vi "Main.vi"() -> ()   [LabVIEW 2015]
doc: "This template is for the Queued Message Handler design pattern.\n\nThe Event Handling Loop generates messages based on user interface actions.\n\nThe Message Handling Loop processes messages generated by the Event Handling Loop, or by other messages. The messages are string values, so new messages can be added easily to the Message Cases case structure in the Message Handling Loop. Each message cluster can also provide an optional value for Message Data, which is a variant that can be converted to whatever message-specific data is required."
uses:
  support/Type Definitions/UI Data.ctl
  support/Status Logger/Status Log.ctl
  TCP/TypeDefs/TCP Data.ctl
  <vilib>/Utility/error.llb/DialogType.ctl
  DAQ/TypeDefs/DAQ data.ctl
  support/Message Queue/Enqueue Message (Single).vi
  support/Global names.vi
  <vilib>/Utility/error.llb/Error Cluster From Error Code.vi
  <vilib>/ErrorRing/Error Ring.xnode
  support/Message Queue/Message Queue.lvlib
  Support/User Event - EHL Stop/User Event - EHL Stop.lvlib
  Model/Model.lvlib
  DAQ/DAQ.lvlib
  PLC/PLC.lvlib
  Logger/Logger.lvlib
  TCP/TCP.lvlib
panel:
  out "Power status":bool
  in  "Remote":bool
  in  "Abort":bool
  in  "Stop Line":bool
  in  "Start Line":bool
  out "Status":string
  in  "Tab Control":T1(tab)
  in  "Power switch":bool
  in  "Positon":dbl(slide) scale=0.0..20.0
  in  "Dispose":bool
  in  "Pump":bool
  in  "Flow [l/s]":dbl=10.0
  in  "Potentiometer (AI)":tag
  in  "LED (DO)":tag
  in  "Bistable switch (DI)":tag
  in  "Monostable switch (DI)":tag
  in  "Send":bool
  in  "Command to send":string
  out "Commands received":string
  in  "Disconnect":bool
  in  "Connect":bool
  out "Connected?":bool
  in  "Type":enum16{"Server", "Client"}(ring)
  in  "Port":u16
  in  "IP":string
  out "Current machine IP":string
  in  "Current printer":u16(ring) items=["PDFCreator", "OKI DATA CORP C5950 kolor (C-2 218)", "Microsoft XPS Document Writer", "Microsoft Print to PDF", "HP LaserJet Professional P1606dn B&W (M3)", "hp LaserJet 1320 PCL 5 B&W (C-2 307)", "Fax", "Canon MP560 KOLOR (DOM)", "Brother PC-FAX v.3.2", "Brother MFC-L8850CDW KOLOR (M6)", "Brother MFC-L2740DW B&W (M6)", "Brother MFC-L2740DW B&W (M3)", "Brother DCP-9020CDW (Dziekan)"]
  in  "Check printers":bool
  in  "Print report":bool
  in  "TDMS View":bool
  in  "Exit":bool
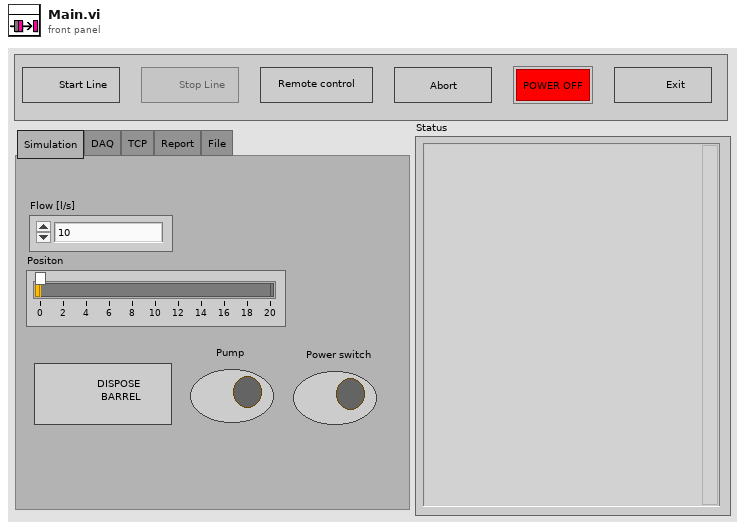
[diagram p1: front panel]
types:
  T1 = enum32{"Simulation", "DAQ", "TCP", "Report", "File"}
  T2 = typedef "Status Log.ctl" = enum16{"Close file", "Open Status file", "Add Status", "Show Status File"}
  T3 = typedef "UI Data.ctl" = cluster{"Start Line Ref":refnum<vi>, "Stop Line Ref":refnum<vi>, "Data Display Ref":refnum<vi>, "Exit Button Ref":refnum<vi>, "Pump Ref":refnum<vi>, "Dispose Ref":refnum<vi>, "Flow Ref":refnum<vi>, "Position Ref":refnum<vi>, "Tab Ref":refnum<vi>, "Print report":refnum<vi>, "Remote":refnum<vi>, "Connection status":refnum<vi>, "Abort":refnum<vi>, "Power status":refnum<vi>, "Power switch":refnum<vi>}
  T4 = typedef "Notifiers.lvlib/Notifiers.ctl" = cluster{"PLC":refnum<notifier>, "Model":refnum<notifier>, "DAQ":refnum<notifier>, "Log":refnum<notifier>, "TCP":refnum<notifier>}
  T5 = typedef "Message Queue.lvlib/All Message Queues.ctl" = cluster{"UI":refnum<queue>, "Model":refnum<queue>, "DAQ":refnum<queue>, "PLC":refnum<queue>, "Log":refnum<queue>, "TCP":refnum<queue>}
  T6 = typedef "TCP.lvlib/TCP Data.ctl" = cluster{"Type":enum16{"Server", "Client"}, "IP":string, "Port":u16, "connection ID":refnum<k5>, "Connected?":bool, "Data":string}
  T7 = typedef "DialogType.ctl" = u16
  T8 = typedef "DAQ.lvlib/DAQ data.ctl" = cluster{"Power switch (DI)":cluster{"Channel":tag, "Data":bool}, "Dispose barrel (DI)":cluster{"Channel":tag, "Data":bool}, "Pump status (DO)":cluster{"Channel":tag, "Data":bool}, "Barrel position (AI)":cluster{"Channel":tag, "Data":dbl}}
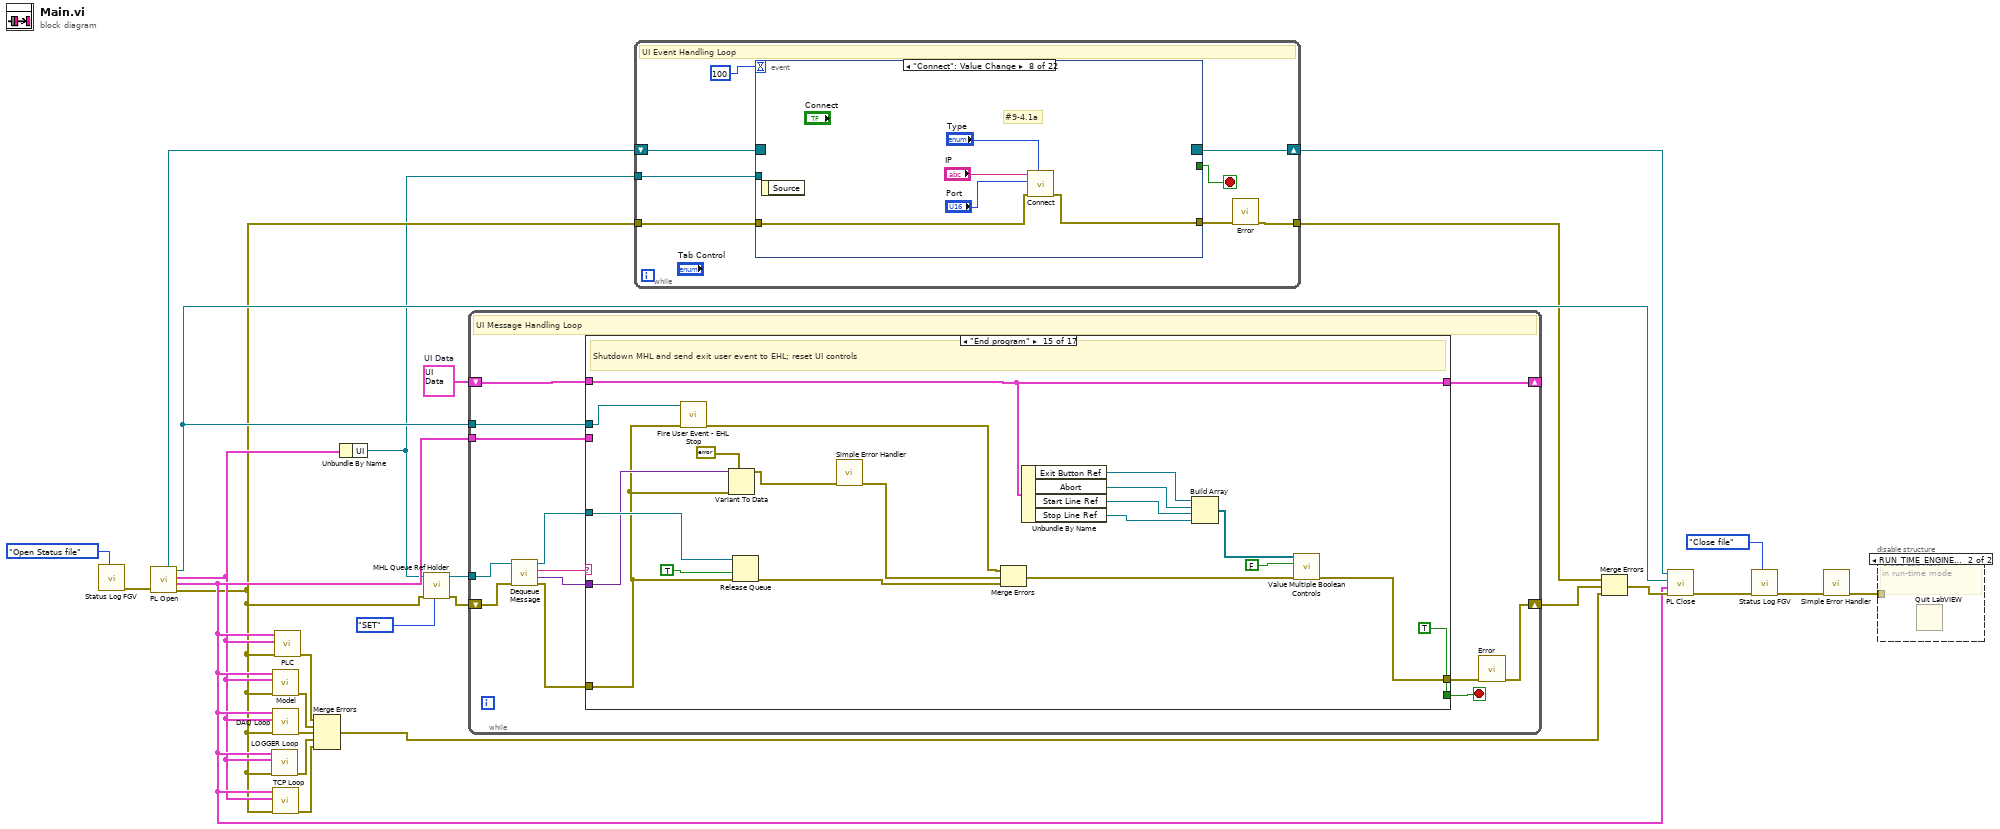
[diagram p0: block diagram]
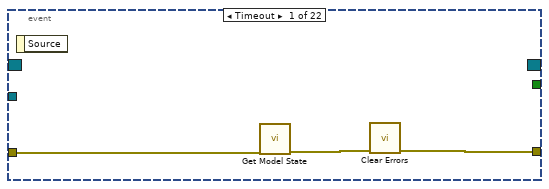
[diagram p2: hidden frame]
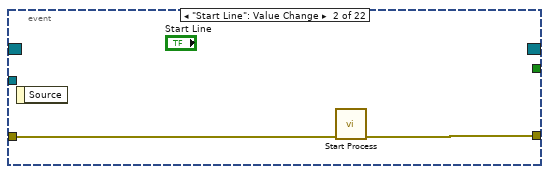
[diagram p3: hidden frame]
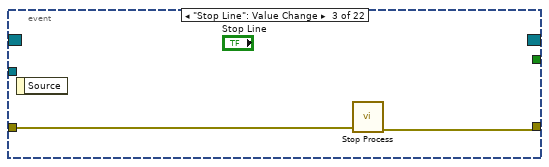
[diagram p4: hidden frame]
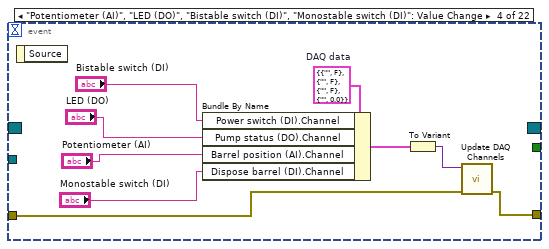
[diagram p5: hidden frame]
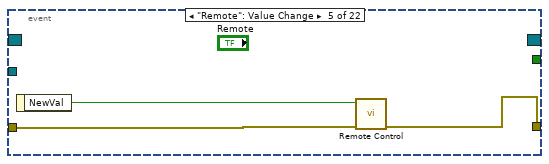
[diagram p6: hidden frame]
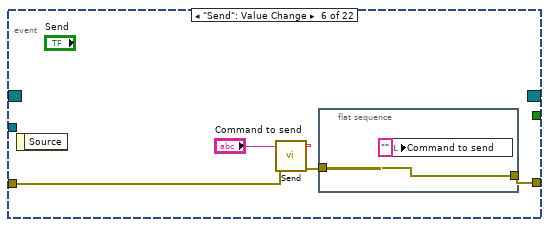
[diagram p7: hidden frame]
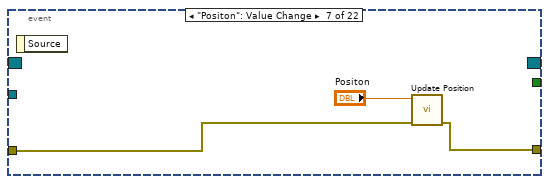
[diagram p8: hidden frame]
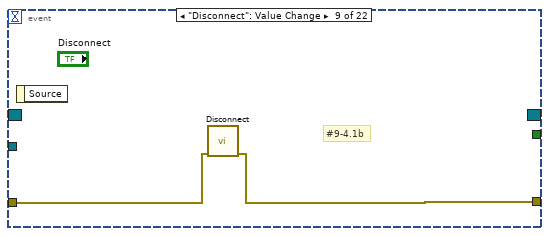
[diagram p9: hidden frame]
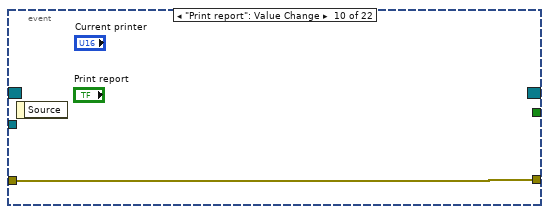
[diagram p10: hidden frame]
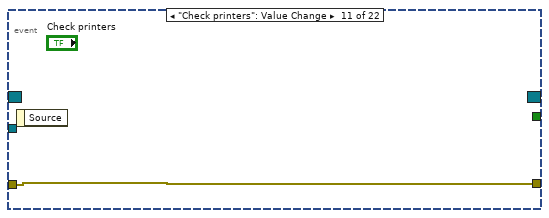
[diagram p11: hidden frame]
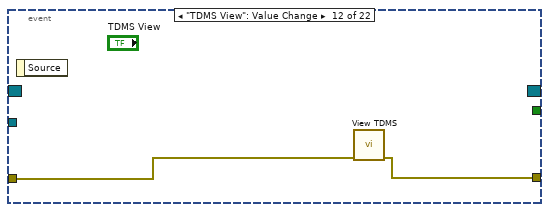
[diagram p12: hidden frame]
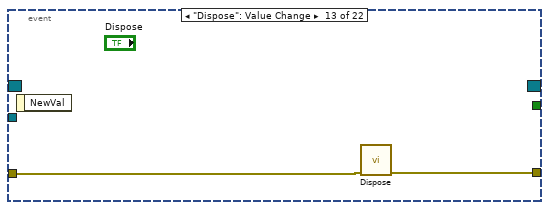
[diagram p13: hidden frame]
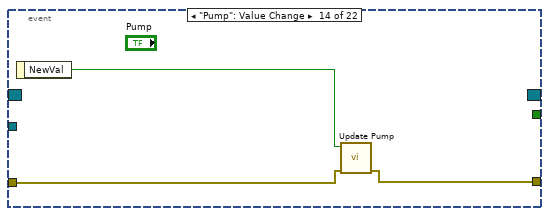
[diagram p14: hidden frame]
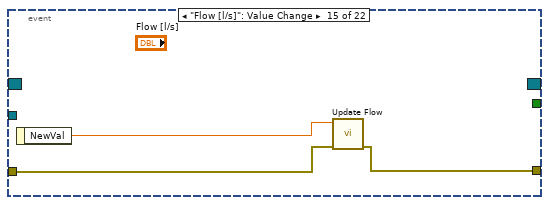
[diagram p15: hidden frame]
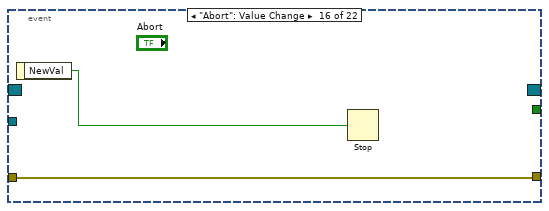
[diagram p16: hidden frame]
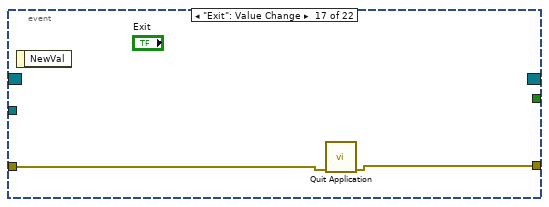
[diagram p17: hidden frame]
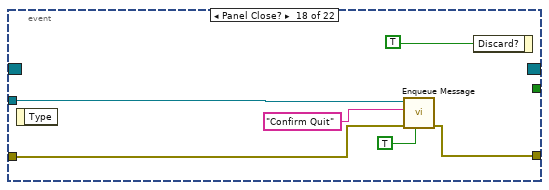
[diagram p18: hidden frame]
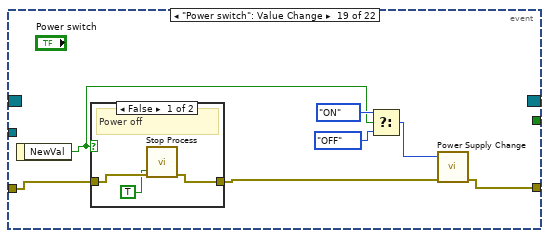
[diagram p19: hidden frame]
diagram:
  w25 = T3 {"Start Line Ref"=refnum, "Stop Line Ref"=refnum, "Data Display Ref"=refnum, "Exit Button Ref"=refnum, "Pump Ref"=refnum, "Dispose Ref"=refnum, "Flow Ref"=refnum, "Position Ref"=refnum, "Tab Ref"=refnum, "Print report"=refnum, "Remote"=refnum, "Connection status"=refnum, "Abort"=refnum, "Power status"=refnum, "Power switch"=refnum}  # UI Data
  n1 = call "Status Log FGV.vi"("Action"=Status_Log."Open Status file") -> ("error out"=w20:errorcluster)  [unwired: 10 in]
  n2 = call "PL Open.vi"("error in"=w20) -> ("error out"=w4:errorcluster, "Notifiers"=w13:T4, "Queues"=w12:T5, "User Event"=w23:refnum<user-event>, "Event Registration Refnum"=w15:refnum<event-registration>)  [unwired: 6 in]
  n3 = call "LOGGER Loop.vi"("error in"=w4, "Queues"=w12, "Notifiers"=w13) -> ("error out"=w8:errorcluster)  [unwired: 8 in]
  n4 = call "Model.vi"("error in"=w4, "Queues"=w12, "Notifiers"=w13) -> ("error out"=w10:errorcluster)  [unwired: 8 in]
  n5 = call "DAQ Loop.vi"("error in"=w4, "Queues"=w12, "Notifiers"=w13) -> ("error out"=w9:errorcluster)  [unwired: 8 in]
  n6 = call "TCP Loop.vi"("error in"=w4, "Queues"=w12, "Notifiers"=w13) -> ("error out"=w7:errorcluster)  [unwired: 8 in]
  n7 = call "PLC.vi"("error in"=w4, "Message Queues"=w12, "Notifiers"=w13) -> ("error out"=w11:errorcluster)  [unwired: 8 in]
  n8 = Merge Errors(w11, w10, w9, w8, w7) -> (w6:errorcluster)
  n9 = Unbundle By Name(w12) -> ("UI"=w1:refnum<queue>)
  n10 = call "MHL Queue Ref Holder.vi"("Action"=enum16{"GET", "SET"}."SET", "error in"=w4, "Message Queue In"=w1) -> ("error out"=w3:errorcluster, "Input Message Queue"=w5:refnum<queue>)  [unwired: 7 in]
  n11 = while {
    shift-right: [w38] -> _
    shift-left: w25 -> [w39]
    tunnel: w23 -> [w36]
    tunnel: w13 -> [w32]
    shift-right: [w28] -> w19
    shift-left: w3 -> [w35]
    tunnel: w5 -> [w30]
    stop <- w37 stop-if-true
    # "UI Message Handling Loop"
    n12 = call "Dequeue Message.vi"("error in (no error)"=w35, "Message Queue"=w30) -> ("error out"=w34:errorcluster, "Message Data"=w31:variant, "Message"=w27:string, "dup Message Queue"=w33:refnum<queue>)  [unwired: 6 in]
    n13 = case "Message Cases" shown="\"End program\"" w27 {
      selector: w27 -> [_ _ _ _ _ _ _ _ _ _ _ _ _ _ _ _ w281]
      tunnel: w33 -> [w41 _ _ _ _ _ _ _ _ _ _ _ w227 w233 w269 _ _]
      tunnel: w34 -> [w42 w48 w71 w106 w121 w140 w158 w160 w176 w188 w216 w219 w228 w235 w252 w276 _]
      tunnel: [w40 w48 w81 w107 w120 w142 w154 w161 w177 w182 w212 w218 w225 w232 w256 w270 w280] -> w29
      tunnel: w39 -> [w43 w62 w92 w108 w127 w152 w153 w167 w180 w181 w194 w223 w229 w239 w261 w275 w282]
      tunnel: [w43 w49 w92 w108 w127 w152 w153 w167 w180 w181 w194 w223 w229 w239 w261 w275 w282] -> w38
      tunnel: [_ _ _ _ _ _ _ _ _ _ _ _ _ _ TRUE _ _] -> w37
      tunnel: w31 -> [_ _ _ _ _ _ w157 w171 w174 w187 w215 w222 _ _ w263 _ _]
      tunnel: w36 -> [_ _ _ _ _ _ _ _ _ _ _ _ _ _ w266 _ _]
      tunnel: w32 -> [_ _ _ _ _ _ _ _ _ _ _ _ _ w238 _ _ _]
      frame "Initialize" {
        w44 = string[] ["Initialize references", "Initialize controls", "Initialize PLC"]  # Message
        # "Prepare application initialization procedure"
        n14 = call "Enqueue Message (Array).vi"("error in (no error)"=w42, "Message Array"=w44, "Message Queue"=w41) -> ("error out"=w40:errorcluster)  [unwired: 7 in, 1 out]
      }
      frame "Initialize references" {
        # "Link references to UI objects"
        n15 = control-ref of="Power switch"() -> (w45:refnum<vi>)
        n16 = control-ref of="Stop Line"() -> (w59:refnum<vi>)
        n17 = control-ref of="Flow [l/s]"() -> (w56:refnum<vi>)
        n18 = control-ref of="Dispose"() -> (w57:refnum<vi>)
        n19 = control-ref of="Exit"() -> (w61:refnum<vi>)
        n20 = control-ref of="Start Line"() -> (w60:refnum<vi>)
        n21 = control-ref of="Pump"() -> (w58:refnum<vi>)
        n22 = Bundle By Name(cluster=w62, "Exit Button Ref"=w61, "Start Line Ref"=w60, "Stop Line Ref"=w59, "Pump Ref"=w58, "Dispose Ref"=w57, "Flow Ref"=w56, "Power switch"=w45) -> (w55:T3)
        n23 = control-ref of="Tab Control"() -> (w53:refnum<vi>)
        n24 = control-ref of="Remote"() -> (w51:refnum<vi>)
        n25 = control-ref of="Connection status"() -> (w50:refnum<vi>)
        n26 = control-ref of="Positon"() -> (w54:refnum<vi>)
        n27 = control-ref of="Print report"() -> (w52:refnum<vi>)
        n28 = control-ref of="Power status"() -> (w46:refnum<vi>)
        n29 = control-ref of="Abort"() -> (w47:refnum<vi>)
        n30 = Bundle By Name(cluster=w55, "Position Ref"=w54, "Tab Ref"=w53, "Print report"=w52, "Remote"=w51, "Connection status"=w50, "Abort"=w47, "Power status"=w46) -> (w49:T3)
      }
      frame "Initialize controls" {
        w80 = "" ("Data received")
        w63 = TRUE ("Enabled")
        w64 = FALSE ("Enabled")
        # "Initialize activity and values of UI objects"
        n31 = Unbundle By Name(w92) -> ("Stop Line Ref"=w105:refnum<vi>, "Print report"=w87:refnum<vi>)
        n32 = Current VI's Menubar() -> (w66:refnum<k9>)
        n33 = Build Array(w105, w87) -> (w104:refnum<vi>[])
        n34 = call "Enable Multiple Controls.vi"("error in"=w71, "Enabled"=w64, "References"=w104) -> ("error out"=w101:errorcluster)  [unwired: 8 in]
        n35 = Set Menu Item Info(7:"Stop" ("item tag"), 8:w71, 9:w64, 11:w66) -> (0:w69:errorcluster, 3:w65:refnum<k9>)  [unwired: 3 in]
        n36 = Unbundle By Name(w92) -> ("Exit Button Ref"=w103:refnum<vi>, "Start Line Ref"=w102:refnum<vi>)
        n37 = call "Power Supply Change.vi"("error in"=w71, "Power status"=enum16{"OFF", "ON"}."OFF") -> ("error out"=w77:errorcluster)  [unwired: 9 in]
        n38 = Build Array(w103, w102) -> (w100:refnum<vi>[])
        n39 = call "Enable Multiple Controls.vi"("error in"=w101, "Enabled"=w63, "References"=w100) -> ("error out"=w95:errorcluster)  [unwired: 8 in]
        n40 = Set Menu Item Info(7:"Start" ("item tag"), 8:w69, 9:w63, 11:w65) -> (0:w67:errorcluster)  [unwired: 3 in, 1 out]
        n41 = Unbundle By Name(w92) -> ("Exit Button Ref"=w99:refnum<vi>, "Start Line Ref"=w98:refnum<vi>, "Stop Line Ref"=w97:refnum<vi>, "Pump Ref"=w96:refnum<vi>, "Remote"=w86:refnum<vi>, "Connection status"=w85:refnum<vi>, "Abort"=w84:refnum<vi>, "Power status"=w83:refnum<vi>, "Power switch"=w73:refnum<vi>)
        n42 = call "Status Display.vi"("Action"=enum16{"Update", "Clear"}."Clear", "error in"=w77) -> ("error out"=w76:errorcluster, "Status"=w74:string)  [unwired: 8 in]
        n43 = local write "Status"(w74) -> ()
        n44 = Build Array(w99, w98, w97, w96, w86, w85, w84, w83, w73) -> (w93:refnum<vi>[])
        n45 = call "Value Multiple Boolean Controls.vi"("error in"=w95, "Value"=FALSE ("Enabled"), "References"=w93) -> ("error out"=w91:errorcluster)  [unwired: 8 in]
        n46 = Unbundle By Name(w92) -> ("Position Ref"=w90:refnum<vi>)
        n47 = Build Array(w90) -> (w89:refnum<vi>[])
        n48 = call "Value Multiple Numeric Controls.vi"("error in"=w91, "Value"=0.0, "References"=w89) -> ("error out"=w79:errorcluster)  [unwired: 8 in]
        n49 = local write "Commands received"(w80) -> ()
        n50 = local write "Command to send"(w80) -> ()
        n51 = call "Update Display.vi"("error in"=w79, "Message string"="UI initialized") -> ("error out"=w68:errorcluster)  [unwired: 9 in]
        n52 = Merge Errors(w68, w67, w76) -> (w81:errorcluster)
      }
      frame "Initialize PLC" {
        # "Initialize Production Line Controller"
        n53 = call "Initialize.vi"("error in"=w106) -> ("error out"=w107:errorcluster)  [unwired: 10 in]
      }
      frame "Start process" {
        w112 = TRUE ("Enabled")
        w116 = FALSE ("Enabled")
        # "Starts process: start PLC, open logger file, create reports files, enable/disable UI controls and update status display"
        n54 = Unbundle By Name(w127) -> ("Exit Button Ref"=w109:refnum<vi>, "Start Line Ref"=w122:refnum<vi>, "Stop Line Ref"=w126:refnum<vi>)
        n55 = Build Array(w109, w122) -> (w128:refnum<vi>[])
        n56 = Build Array(w126) -> (w125:refnum<vi>[])
        n57 = call "Start.vi"("error in"=w121) -> ("error out"=w124:errorcluster)  [unwired: 10 in]
        n58 = call "Enable Multiple Controls.vi"("error in"=w121, "Enabled"=w112, "References"=w125) -> ("error out"=w114:errorcluster)  [unwired: 8 in]
        n59 = call "Enable Multiple Controls.vi"("error in"=w121, "Enabled"=w116, "References"=w128) -> ("error out"=w118:errorcluster)  [unwired: 8 in]
        n60 = global read "Global names.vi" "Starting"() -> (w110:string)
        n61 = Current VI's Menubar() -> (w111:refnum<k9>)
        n62 = call "Update Display.vi"("error in"=w124, "Message string"=w110) -> ("error out"=w123:errorcluster)  [unwired: 9 in]
        n63 = Set Menu Item Info(7:"Start" ("item tag"), 8:w118, 9:w116, 11:w111) -> (0:w117:errorcluster)  [unwired: 3 in, 1 out]
        n64 = Set Menu Item Info(7:"Stop" ("item tag"), 8:w114, 9:w112, 11:w111) -> (0:w113:errorcluster)  [unwired: 3 in, 1 out]
        n65 = Merge Errors(w123, w117, w113) -> (w120:errorcluster)
      }
      frame "Stop process" {
        w131 = FALSE ("Enabled")
        w132 = TRUE ("Enabled")
        # "Stops process: stop PLC, close logger file, save and close report files, enable/disable UI controls and update status display"
        n66 = Unbundle By Name(w152) -> ("Exit Button Ref"=w129:refnum<vi>, "Start Line Ref"=w145:refnum<vi>, "Stop Line Ref"=w151:refnum<vi>)
        n67 = call "Stop.vi"("error in"=w140) -> ("error out"=w147:errorcluster)  [unwired: 10 in]
        n68 = Build Array(w151) -> (w141:refnum<vi>[])
        n69 = Build Array(w129, w145) -> (w149:refnum<vi>[])
        n70 = global read "Global names.vi" "Stopping"() -> (w130:string)
        n71 = Build Array (concatenate)(w149, w141) -> (w148:refnum<vi>[])
        n72 = call "Enable Multiple Controls.vi"("error in"=w140, "Enabled"=w132, "References"=w149) -> ("error out"=w137:errorcluster)  [unwired: 8 in]
        n73 = call "Enable Multiple Controls.vi"("error in"=w140, "Enabled"=w131, "References"=w141) -> ("error out"=w144:errorcluster)  [unwired: 8 in]
        n74 = call "Value Multiple Boolean Controls.vi"("error in"=w140, "Value"=FALSE, "References"=w148) -> ("error out"=w143:errorcluster)  [unwired: 8 in]
        n75 = call "Update Display.vi"("error in"=w147, "Message string"=w130) -> ("error out"=w146:errorcluster)  [unwired: 9 in]
        n76 = Current VI's Menubar() -> (w138:refnum<k9>)
        n77 = Set Menu Item Info(7:"Start" ("item tag"), 8:w137, 9:w132, 11:w138) -> (0:w135:errorcluster, 3:w133:refnum<k9>)  [unwired: 3 in]
        n78 = Set Menu Item Info(7:"Stop" ("item tag"), 8:w135, 9:w131, 11:w133) -> (0:w134:errorcluster)  [unwired: 3 in, 1 out]
        n79 = Merge Errors(w146, w134, w144, w143) -> (w142:errorcluster)
      }
      frame "Update IP" {
        # "Update IP address of current machine"
        n80 = Variant To Data(error in=w158, type="", Variant=w157) -> (data=→"Current machine IP":string, error out=w154:errorcluster)
      }
      frame "Update display" {
        # "Updates status display, status log file and word report file"
        n81 = Variant To Data(error in=w160, type="", Variant=w171) -> (data=w159:string, error out=w164:errorcluster)
        n82 = call "Status Display.vi"("Action"=enum16{"Update", "Clear"}."Update", "error in"=w164, "Status line"=w159) -> ("error out"=w162:errorcluster, "Status"=→"Status":string)  [unwired: 7 in]
        n83 = call "Status Log FGV.vi"("Action"=Status_Log."Add Status", "error in"=w164, "Status"=w159) -> ("error out"=w163:errorcluster)  [unwired: 8 in]
        n84 = property on="Status" class="Str"("Text.Scroll Position"=-1) -> ()  [unwired: 2 in, 2 out]
        n85 = Merge Errors(w163, w162) -> (w161:errorcluster)
      }
      frame "Update position" {
        # "Programmatically update position of the barrel slider"
        n86 = Variant To Data(error in=w176, type=0.0 ("Value"), Variant=w174) -> (data=w172:dbl, error out=w175:errorcluster)
        n87 = Unbundle By Name(w180) -> ("Position Ref"=w179:refnum<vi>)
        n88 = Build Array(w179) -> (w178:refnum<vi>[])
        n89 = call "Value Multiple Numeric Controls.vi"("error in"=w175, "Value"=w172, "References"=w178) -> ("error out"=w177:errorcluster)  [unwired: 8 in]
      }
      frame "Update Connection UI" {
        w186 = T6 {"Type"=enum."Server", "IP"="", "Port"=0, "connection ID"=refnum, "Connected?"=FALSE, "Data"=""}  # TCP Data
        # "Updates TCP conection UI indicators"
        n90 = Variant To Data(error in=w188, type=w186, Variant=w187) -> (data=w185:T6, error out=w182:errorcluster)
        n91 = Unbundle By Name(w185) -> ("Connected?"=→"Connected?":bool, "Data"=→"Commands received":string)
      }
      frame "Power status change" {
        # "Update main switch LED and Start/Stop buttons according to power status change (DAQ DI)"
        n92 = Variant To Data(error in=w216, type=TRUE, Variant=w215) -> (data=w195:bool, error out=w199:errorcluster)
        "Power status" <- w195
        n93 = Unbundle By Name(w194) -> ("Position Ref"=w189:refnum<vi>, "Dispose Ref"=w193:refnum<vi>, "Pump Ref"=w192:refnum<vi>)
        n94 = Unbundle By Name(w194) -> ("Start Line Ref"=w191:refnum<vi>, "Stop Line Ref"=w213:refnum<vi>)
        n95 = Build Array(w189, w193, w192, w191) -> (w190:refnum<vi>[])
        n96 = Build Array(w191) -> (w211:refnum<vi>[])
        n97 = Build Array(w213) -> (w208:refnum<vi>[])
        n98 = Build Array (concatenate)(w211, w208) -> (w210:refnum<vi>[])
        n99 = Current VI's Menubar() -> (w202:refnum<k9>)
        n100 = call "Enable Multiple Controls.vi"("error in"=w199, "Enabled"=w195, "References"=w190) -> ("error out"=w206:errorcluster)  [unwired: 8 in]
        n101 = Set Menu Item Info(7:"Start" ("item tag"), 8:w199, 9:w195, 11:w202) -> (0:w200:errorcluster, 3:w196:refnum<k9>)  [unwired: 3 in]
        n102 = call "Value Multiple Boolean Controls.vi"("error in"=w199, "Value"=FALSE, "References"=w210) -> ("error out"=w205:errorcluster)  [unwired: 8 in]
        n103 = call "Enable Multiple Controls.vi"("error in"=w199, "Enabled"=FALSE, "References"=w208) -> ("error out"=w204:errorcluster)  [unwired: 8 in]
        n104 = Set Menu Item Info(7:"Stop" ("item tag"), 8:w200, 9:FALSE ("enabled"), 11:w196) -> (0:w197:errorcluster)  [unwired: 3 in, 1 out]
        n105 = Merge Errors(w206, w205, w204, w197) -> (w212:errorcluster)
      }
      frame "Error" {
        w217 = T7 2 items=["no dialog", "OK message", "continue or stop message", "OK message + warnings", "continue/stop + warnings"] ("type of dialog (OK msg:1)")
        # "Display error dialog box and quit application"
        n106 = Variant To Data(error in=w219, type=errorcluster {"status"=FALSE, "code"=0, "source"=""} ("error constant"), Variant=w222) -> (data=w220:errorcluster, error out=w218:errorcluster)
        n107 = call <vilib>:"Simple Error Handler.vi"("type of dialog (OK msg:1)"=w217, "error in (no error)"=w220) -> ()  [unwired: 3 in, 5 out]
      }
      frame "Exit" {
        # "Start exit procedure: stop PLC, then send Exit message to PLC and go to PLC confirmation loop"
        n108 = Flush Queue(queue=w227, error in (no error)=w228) -> (error out=w224:errorcluster)  [unwired: 2 out]
        n109 = call "Exit PLC.vi"("error in"=w224) -> ("error out"=w226:errorcluster)  [unwired: 10 in]
        n110 = call "Wait on PLC Exit.vi"("error in"=w226) -> ("error out"=w225:errorcluster)  [unwired: 10 in]
      }
      frame "Wait on PLC exit" {
        # "Wait until PLC shutdown"
        n111 = Unbundle By Name(w238) -> ("PLC"=w237:refnum<notifier>)
        n112 = Wait on Notification(notifier=w237, timeout in ms (-1)=10, error in (no error)=w235) -> (notification=w231:string, timed out?=w234:bool, error out=w230:errorcluster)  [unwired: 1 in, 1 out]
        n113 = case shown="False" w234 {
          tunnel: [w240 w249] -> w232
          tunnel: w230 -> [w241 w246]
          tunnel: w233 -> [_ w247]
          tunnel: w231 -> [_ w242]
          frame True {
            # "Shutdown notification from PLC not received"
            n114 = call "Wait on PLC Exit.vi"("error in"=w241) -> ("error out"=w240:errorcluster)  [unwired: 10 in]
          }
          frame False {
            # "Shutdown notification from PLC received (handshake)"
            n115 = call "Update Display.vi"("error in"=w246, "Message string"=w242) -> ("error out"=w245:errorcluster)  [unwired: 9 in]
            n116 = call "Update Display.vi"("error in"=w245, "Message string"="Application quits" ("Message")) -> ("error out"=w244:errorcluster)  [unwired: 9 in]
            n117 = call-poly "Enqueue Message.vi"("error in (no error)"=w244, "Message"="End program", "Message Queue"=w247) -> ("error out"=w249:errorcluster)  [unwired: 7 in, 1 out]
          }
        }
      }
      frame "End program" {
        # "Shutdown MHL and send exit user event to EHL; reset UI controls"
        n118 = call "Fire User Event - EHL Stop.vi"("error in (no error)"=w252, "User Event - Stop"=w266) -> ("error out"=w251:errorcluster)  [unwired: 9 in]
        n119 = Variant To Data(error in=w252, type=errorcluster {"status"=FALSE, "code"=0, "source"=""} ("error constant"), Variant=w263) -> (data=w264:errorcluster)  [unwired: 1 out]
        n120 = Release Queue(queue=w269, force destroy? (F)=TRUE, error in (no error)=w252) -> (error out=w267:errorcluster)  [unwired: 2 out]
        n121 = call <vilib>:"Simple Error Handler.vi"("error in (no error)"=w264) -> ("error out"=w250:errorcluster)  [unwired: 4 in, 4 out]
        n122 = Merge Errors(w251, w250, w267) -> (w257:errorcluster)
        n123 = Unbundle By Name(w261) -> ("Exit Button Ref"=w260:refnum<vi>, "Abort"=w255:refnum<vi>, "Start Line Ref"=w254:refnum<vi>, "Stop Line Ref"=w253:refnum<vi>)
        n124 = Build Array(w260, w255, w254, w253) -> (w259:refnum<vi>[])
        n125 = call "Value Multiple Boolean Controls.vi"("error in"=w257, "Value"=FALSE, "References"=w259) -> ("error out"=w256:errorcluster)  [unwired: 8 in]
      }
      frame "Confirm Quit" {
        # "Confirm Quit - Message that can confirm whether or not the user wants to exit the application."
        n126 = Two Button Dialog(message="Are you sure?", 1:"Continue" ("F button name (\"Cancel\")"), 2:"Quit" ("T button name (\"OK\")")) -> (T button?=w271:bool)
        n127 = case shown="True" w271 {
          tunnel: w276 -> [w277 w279]
          tunnel: [w277 w278] -> w270
          frame False {
          }
          frame True {
            n128 = call "Quit Application.vi"("error in"=w279) -> ("error out"=w278:errorcluster)  [unwired: 10 in]
          }
        }
      }
      frame Default {
        # "Incorrect message: show error and clear error"
        n129 = xnode "Error Ring"("parameter 0"=w281) -> ("error out"=w280:errorcluster)
      }
    }
    n130 = call "Error.vi"("error in"=w29) -> ("error out"=w28:errorcluster)  [unwired: 10 in]
  }
  n131 = while {
    tunnel: w1 -> [w292]
    shift-right: [w296] -> w26
    shift-left: w15 -> [w297]
    tunnel: [w290] -> w14
    tunnel: w4 -> [w293]
    stop <- w295 stop-if-true
    # "UI Event Handling Loop"
    n132 = event shown="[7] \"Connect\": Value Change" {
      selector: w297 -> [_ _ _ _ _ _ _ _ _ _ _ _ _ _ _ _ _ _ _ _ _ _]
      dyn-events: [_ _ _ _ _ _ _ _ _ _ _ _ _ _ _ _ _ _ _ _ _ _] -> w296
      timeout: 100 -> [_ _ _ _ _ _ _ _ _ _ _ _ _ _ _ _ _ _ _ _ _ _]
      tunnel: [_ _ _ _ _ _ _ _ _ _ _ _ _ _ _ _ _ _ _ _ TRUE ("Discard?") _] -> w295
      tunnel: w292 -> [_ _ _ _ _ _ _ _ _ _ _ _ _ _ _ _ _ w354 _ _ _ _]
      tunnel: [w298 w301 w303 w313 w316 w317 w324 w326 w331 w333 w334 w335 w337 w340 w343 w346 w347 w353 w355 w366 w367 w370] -> w291
      tunnel: w293 -> [w300 w302 w304 w312 w315 w318 w323 w327 w332 w333 w334 w336 w338 w341 w344 w346 w348 w349 w357 w366 w367 w369]
      event Timeout {
        n133 = event-data() -> ()  [unwired: 1 in, 1 out]
        n134 = call "Get Model State.vi"("error in (no error)"=w300) -> ("error out"=w299:errorcluster)  [unwired: 10 in]
        n135 = call <vilib>:"Clear Errors.vi"("error in (no error)"=w299) -> ("error out"=w298:errorcluster)  [unwired: 5 in, 1 out]
      }
      event "Start Line": Value Change {
        n136 = event-data() -> ()  [unwired: 1 in, 1 out]
        n137 = call "Start Process.vi"("error in"=w302) -> ("error out"=w301:errorcluster)  [unwired: 10 in]
      }
      event "Stop Line": Value Change {
        n138 = event-data() -> ()  [unwired: 1 in, 1 out]
        n139 = call "Stop Process.vi"("error in"=w304) -> ("error out"=w303:errorcluster)  [unwired: 10 in]
      }
      event "Potentiometer (AI)", "LED (DO)", "Bistable switch (DI)", "Monostable switch (DI)": Value Change {
        w306 = T8 {"Power switch (DI)"={"Channel"="", "Data"=FALSE}, "Dispose barrel (DI)"={"Channel"="", "Data"=FALSE}, "Pump status (DO)"={"Channel"="", "Data"=FALSE}, "Barrel position (AI)"={"Channel"="", "Data"=0.0}}  # DAQ data
        n140 = event-data() -> ()  [unwired: 1 in, 1 out]
        n141 = Bundle By Name(cluster=w306, "Power switch (DI).Channel"="Bistable switch (DI)", "Pump status (DO).Channel"="LED (DO)", "Barrel position (AI).Channel"="Potentiometer (AI)", "Dispose barrel (DI).Channel"="Monostable switch (DI)") -> (w309:T8)
        n142 = To Variant(anything=w309) -> (Variant=w305:variant)
        n143 = call "Update DAQ Channels.vi"("error in"=w312, "Message Data"=w305) -> ("error out"=w313:errorcluster)  [unwired: 9 in]
      }
      event "Remote": Value Change {
        n144 = event-data() -> ("NewVal"=w314:bool)  [unwired: 1 in]
        n145 = call "Remote Control.vi"("error in"=w315, "Remote"=w314) -> ("error out"=w316:errorcluster)  [unwired: 9 in]
      }
      event "Send": Value Change {
        n146 = event-data() -> ()  [unwired: 1 in, 1 out]
        n147 = call "Send.vi"("error in"=w318, "Data"="Command to send") -> ("error out"=w319:errorcluster)  [unwired: 9 in]
        n148 = flat-sequence {
          tunnel: w319 -> [w321]
          tunnel: [w321] -> w317
          frame #0 {
            n149 = local write "Command to send"("" ("Data to send")) -> ()
          }
        }
      }
      event "Positon": Value Change {
        n150 = event-data() -> ()  [unwired: 1 in, 1 out]
        n151 = call "Update Position.vi"("error in (no error)"=w323, "Position"="Positon") -> ("error out"=w324:errorcluster)  [unwired: 9 in]
      }
      event "Connect": Value Change {
        # "#9-4.1a"
        n152 = event-data() -> ()  [unwired: 1 in, 1 out]
        n153 = call "Connect.vi"("Type"="Type", "error in"=w327, "Port"="Port", "IP"="IP") -> ("error out"=w326:errorcluster)  [unwired: 7 in]
      }
      event "Disconnect": Value Change {
        # "#9-4.1b"
        n154 = event-data() -> ()  [unwired: 1 in, 1 out]
        n155 = call "Disconnect.vi"("error in"=w332) -> ("error out"=w331:errorcluster)  [unwired: 10 in]
      }
      event "Print report": Value Change {
        n156 = event-data() -> ()  [unwired: 1 in, 1 out]
      }
      event "Check printers": Value Change {
        n157 = event-data() -> ()  [unwired: 1 in, 1 out]
      }
      event "TDMS View": Value Change {
        n158 = event-data() -> ()  [unwired: 1 in, 1 out]
        n159 = call "View TDMS.vi"("error in"=w336) -> ("error out"=w335:errorcluster)  [unwired: 10 in]
      }
      event "Dispose": Value Change {
        n160 = event-data() -> ()  [unwired: 1 in, 1 out]
        n161 = call "Dispose.vi"("error in (no error)"=w338) -> ("error out"=w337:errorcluster)  [unwired: 10 in]
      }
      event "Pump": Value Change {
        n162 = event-data() -> ("NewVal"=w339:bool)  [unwired: 1 in]
        n163 = call "Update Pump.vi"("error in (no error)"=w341, "Pump State"=w339) -> ("error out"=w340:errorcluster)  [unwired: 9 in]
      }
      event "Flow [l/s]": Value Change {
        n164 = event-data() -> ("NewVal"=w342:dbl)  [unwired: 1 in]
        n165 = call "Update Flow.vi"("error in (no error)"=w344, "Flow"=w342) -> ("error out"=w343:errorcluster)  [unwired: 9 in]
      }
      event "Abort": Value Change {
        n166 = event-data() -> ("NewVal"=w345:bool)  [unwired: 1 in]
        n167 = Stop(stop? (T)=w345) -> ()
      }
      event "Exit": Value Change {
        n168 = event-data() -> ()  [unwired: 1 in, 1 out]
        n169 = call "Quit Application.vi"("error in"=w348) -> ("error out"=w347:errorcluster)  [unwired: 10 in]
      }
      event Panel Close? {
        n170 = event-data() -> ()  [unwired: 1 in, 1 out]
        n171 = call-poly "Enqueue Message.vi"("Priority Message? (F)"=TRUE, "error in (no error)"=w349, "Message"="Confirm Quit", "Message Queue"=w354) -> ("error out"=w353:errorcluster)  [unwired: 6 in, 1 out]
        n172 = event-data("Discard?"=TRUE) -> ()  [unwired: 1 in, 1 out]
      }
      event "Power switch": Value Change {
        n173 = event-data() -> ("NewVal"=w358:bool)  [unwired: 1 in]
        n174 = case shown="False" w358 {
          tunnel: w357 -> [w364 w365]
          tunnel: [w363 w365] -> w356
          frame False {
            # "Power off"
            n175 = call "Stop Process.vi"("Priority Message? (F)"=TRUE, "error in"=w364) -> ("error out"=w363:errorcluster)  [unwired: 9 in]
          }
          frame True {
            # "Power on"
          }
        }
        n176 = Select(t=enum16{"OFF", "ON"}."ON" ("Power status"), s=w358, f=enum16{"OFF", "ON"}."OFF" ("Power status")) -> (s? t:f=w359:enum16{"OFF", "ON"})
        n177 = call "Power Supply Change.vi"("error in"=w356, "Power status"=w359) -> ("error out"=w355:errorcluster)  [unwired: 9 in]
      }
      event Application Instance Close {
        n178 = event-data() -> ()  [unwired: 1 in, 1 out]
      }
      event User Event {
        n179 = event-data() -> ()  [unwired: 1 in, 1 out]
      }
      event Menu Selection (User) {
        n180 = event-data() -> ("ItemTag"=w371:string)  [unwired: 1 in]
        n181 = case shown="\"logdir\"" w371 {
          tunnel: [w372 w375 w376 w380 w381 w383] -> w370
          tunnel: w369 -> [w372 w374 w377 w379 w382 w384]
          frame Default {
          }
          frame "logdir" {
            n182 = global read "Global names.vi" "Status log dir"() -> (w373:string)
            n183 = call "Open Dir.vi"("error in"=w374, "dir"=w373) -> ("error out"=w375:errorcluster)  [unwired: 9 in]
          }
          frame "statuslog" {
            n184 = call "Status Log FGV.vi"("Action"=Status_Log."Show Status File", "error in"=w377) -> ("error out"=w376:errorcluster)  [unwired: 9 in]
          }
          frame "Start" {
            n185 = call "Start Process.vi"("error in"=w379) -> ("error out"=w380:errorcluster)  [unwired: 10 in]
          }
          frame "Stop" {
            n186 = call "Stop Process.vi"("error in"=w382) -> ("error out"=w381:errorcluster)  [unwired: 10 in]
          }
          frame "Exit" {
            n187 = call "Quit Application.vi"("error in"=w384) -> ("error out"=w383:errorcluster)  [unwired: 10 in]
          }
        }
      }
    }
    n188 = call "Error.vi"("error in"=w291) -> ("error out"=w290:errorcluster)  [unwired: 10 in]
  }
  n189 = Merge Errors(w14, w19, w6) -> (w18:errorcluster)
  n190 = call "PL Close.vi"("error in"=w18, "Notifiers"=w13, "User Event"=w23, "Event Registration Refnum in"=w26) -> ("error out"=w24:errorcluster)  [unwired: 7 in]
  n191 = call "Status Log FGV.vi"("Action"=Status_Log."Close file", "error in"=w24) -> ("error out"=w16:errorcluster)  [unwired: 9 in]
  n192 = call <vilib>:"Simple Error Handler.vi"("error in (no error)"=w16) -> ("error out"=w17:errorcluster)  [unwired: 4 in, 4 out]
  n193 = disable-structure shown="RUN_TIME_ENGINE==True" {
    disable-tunnel: w17 -> [_ _]
    frame condition #0 (active) {
    }
    frame condition #1 {
      # "Close LabVIEW\nin run-time mode"
      n194 = Quit LabVIEW() -> ()  [unwired: 1 in]
    }
  }
